vi "_Set Item Property.vi"(6 "Set as Binary String":bool=TRUE, 8 "error in (no error)":errorcluster, 9 "Value":variant, 10 "Property Name":string, 11 "Item Ref in":T1 format="%.0x") -> (0 "error out":errorcluster, 3 "Item Ref out":T1 format="%.0x", 4 "Replaced":bool)   [LabVIEW 2020, in "Custom Device Offline API.lvlib"]
uses:
  <vilib>/NI VeriStand/Custom Device Offline API/Custom Device Offline API.lvlib
  <vilib>/NI VeriStand/Custom Device API/Custom Device Item Ref.ctl
  <vilib>/NI VeriStand/Custom Device API/Custom Device API.lvlib
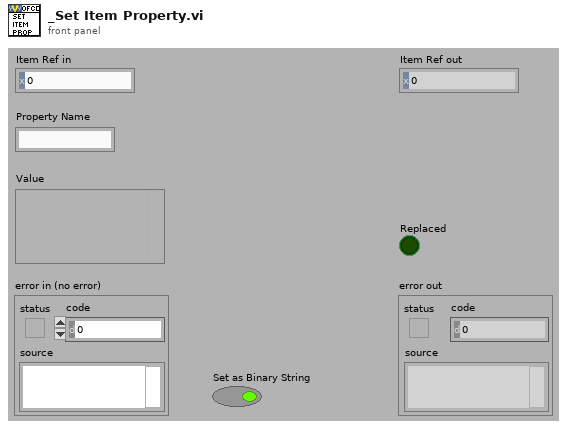
[diagram p1: front panel]
types:
  T1 = typedef "Custom Device API.lvlib/Custom Device Item Ref.ctl" = u64
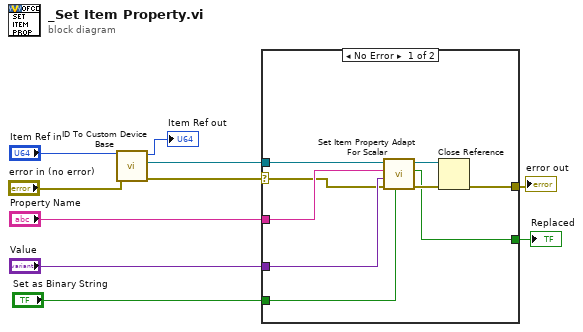
[diagram p0: block diagram]
diagram:
  n1 = call <vilib>:"ID To Custom Device Base.vi"("error in (no error)"="error in (no error)", "ID in"="Item Ref in") -> ("error out"=w8:errorcluster, "BaseNode"=w7:refnum<k24>, "ID out"=→"Item Ref out":u64)  [unwired: 7 in]
  n2 = case shown="No Error" w8 {
    selector: w8 -> [w16 w20]
    tunnel: w7 -> [w19 _]
    tunnel: "Property Name" -> [w18 _]
    tunnel: "Value" -> [w17 _]
    tunnel: [w13 _] -> w2
    tunnel: [w12 w20] -> w3
    tunnel: "Set as Binary String" -> [w11 _]
    frame No Error {
      n3 = call <vilib>:"Set Item Property Adapt For Scalar.vi"("Set String as Binary"=w11, "error in (no error)"=w16, "Value"=w17, "Property Name"=w18, "CDBase"=w19) -> ("error out"=w15:errorcluster, "Replaced"=w13:bool, "CDBase"=w14:refnum<k24>)  [unwired: 4 in]
      n4 = Close Reference(reference=w14, error in (no error)=w15) -> (error out=w12:errorcluster)
    }
    frame Error {
    }
  }
  "error out" <- w3
  "Replaced" <- w2
